vi "HP81110A Output Get.vi"(8 "error in (no error)":errorcluster, 11 "VISA session":refnum<visa-resource-name>) -> (0 "error out":errorcluster, 1 "output2OUT":bool caption="Output 2", 2 "notoutput1OUT":bool caption="Not-Output 1", 3 "dup VISA session":refnum<visa-resource-name>, 4 "notoutput2OUT":bool caption="Not-Output 2", 5 "output1OUT":bool caption="Output 1")   [LabVIEW 2009]
doc: "This VI switches the complement outputs on or off.\n\nNotes:\n\n(1) Available with HP 81112A 3.8V/330MHz output channels."
panel:
  # "On"
  # "Off"
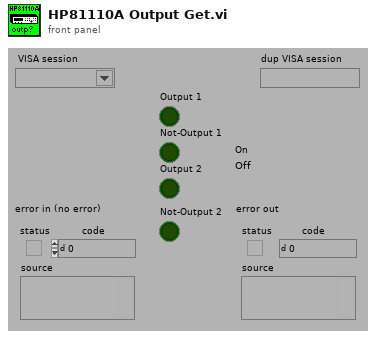
[diagram p1: front panel]
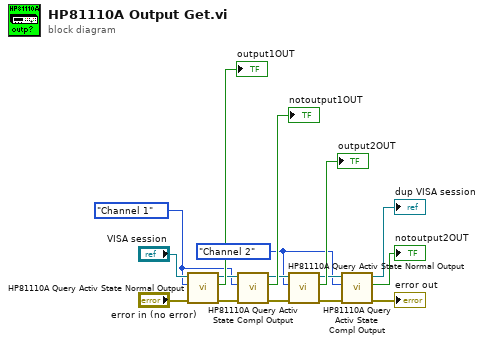
[diagram p0: block diagram]
diagram:
  w1 = enum16{"Invalid", "Channel 1", "Channel 2"}."Channel 2" ("Channel (1:Channel 1)")
  w2 = enum16{"Invalid", "Channel 1", "Channel 2"}."Channel 1" ("Channel (1:Channel 1)")
  n1 = call "HP81110A Query Activ State Normal Output.vi"("error in (no error)"="error in (no error)", "Channel (1:Channel 1)"=w2, "VISA session"="VISA session") -> ("error out"=w10:errorcluster, "Normal State"=→"output1OUT":bool, "dup VISA session"=w9:refnum<visa-resource-name>)  [unwired: 6 out]
  n2 = call "HP81110A Query Activ State Compl Output.vi"("error in (no error)"=w10, "Channel (1:Channel 1)"=w2, "VISA session"=w9) -> ("error out"=w11:errorcluster, "Complement State"=→"notoutput1OUT":bool, "dup VISA session"=w13:refnum<visa-resource-name>)  [unwired: 6 out]
  n3 = call "HP81110A Query Activ State Normal Output.vi"("error in (no error)"=w11, "Channel (1:Channel 1)"=w1, "VISA session"=w13) -> ("error out"=w12:errorcluster, "Normal State"=→"output2OUT":bool, "dup VISA session"=w8:refnum<visa-resource-name>)  [unwired: 6 out]
  n4 = call "HP81110A Query Activ State Compl Output.vi"("error in (no error)"=w12, "Channel (1:Channel 1)"=w1, "VISA session"=w8) -> ("error out"=→"error out":errorcluster, "Complement State"=→"notoutput2OUT":bool, "dup VISA session"=→"dup VISA session":refnum<visa-resource-name>)  [unwired: 6 out]
